vi "RPi_I2C_BME280_read_example.vi"() -> ()   [LabVIEW 2020]
doc: "This example shows how to read the BMP280 sensor by using a Raspberry PI and LabVIEW.\n\nMIT License\nCopyright (c) 2021 Asper"
uses:
  <vilib>/MakerHub/LINX/Public/Utilities/Open Local.vi
  <vilib>/MakerHub/LINX/LMH-LINX.lvlib
panel:
  out "Graph":T1(graph)
  in  "Stop":bool
  out "Last measures":T2
  out "Error Out":errorcluster
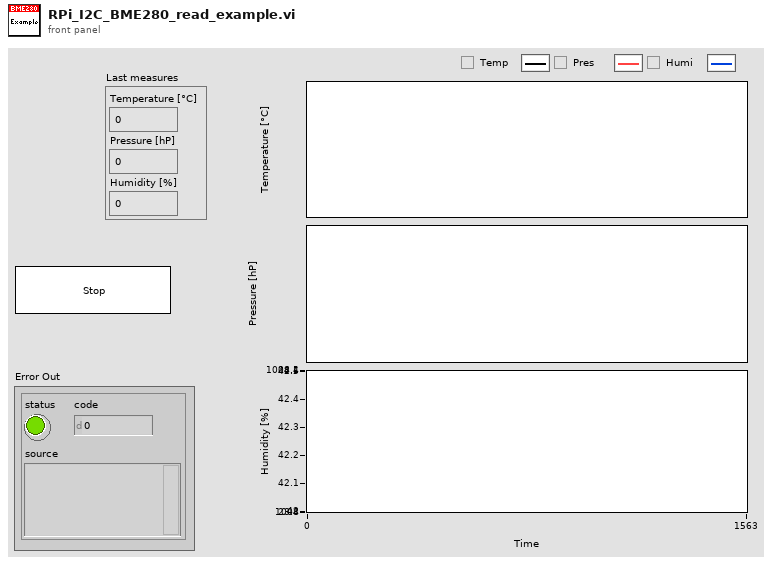
[diagram p1: front panel]
types:
  T1 = cluster{"Temperature":dbl, "Pressure":dbl, "Humidity":dbl}
  T2 = cluster{"Temperature [°C]":dbl, "Pressure [hP]":dbl, "Humidity [%]":dbl}
  T3 = typedef "LMH-LINX.lvlib/LINX Ref.ctl" = cluster{"IO":T4, "Interface":T5, "LINX Device Config":T6}
  T4 = typedef "LMH-LINX.lvlib/Platform.ctl" = enum16{"Remote", "Local"}
  T5 = typedef "LMH-LINX.lvlib/Interface.ctl" = enum16{"Serial", "TCP"}
  T6 = typedef "LMH-LINX.lvlib/Device.lvlib/LINX Device Config.ctl" = cluster{"Interface":T5, "COM Port":refnum<visa-resource-name>, "TCP Configuration":T7, "Device Family":u8, "Device ID":u8, "Device Name":string, "TCP Ref":refnum<k5>, "Channels":T8}
  T7 = typedef "LMH-LINX.lvlib/Device.lvlib/TCP Config.ctl" = cluster{"IP Address":string, "Port":u16}
  T8 = typedef "LMH-LINX.lvlib/Channels.ctl" = cluster{"DI":u8[], "DO":u8[], "AI":u8[], "AO":u8[], "PWM":u8[], "QE":u8[], "UART":u8[], "I2C 2":u8[], "SPI":u8[], "CAN":u8[], "Servo":u8[], "AI Ref (V)":dbl, "AI Resolution (Bits)":u8, "AO Ref (V)":dbl, "AO Resolution (Bits)":u8}
  T9 = typedef "BME280_Calibration_Coefficients.ctl" = cluster{"Temperature":cluster{"dig_T1":u16, "dig_T2":i16, "dig_T3":i16}, "Pressure":cluster{"dig_P1":u16, "dig_P2":i16, "dig_P3":i16, "dig_P4":i16, "dig_P5":i16, "dig_P6":i16, "dig_P7":i16, "dig_P8":i16, "dig_P9":i16}, "Humidity":cluster{"dig_H1":u8, "dig_H2":i16, "dig_H3":u8, "dig_H4":i16, "dig_H5":i16, "dig_H6":i8}}
  T10 = cluster{"pres_raw":u32, "temp_raw":u32, "hum_raw":u32}
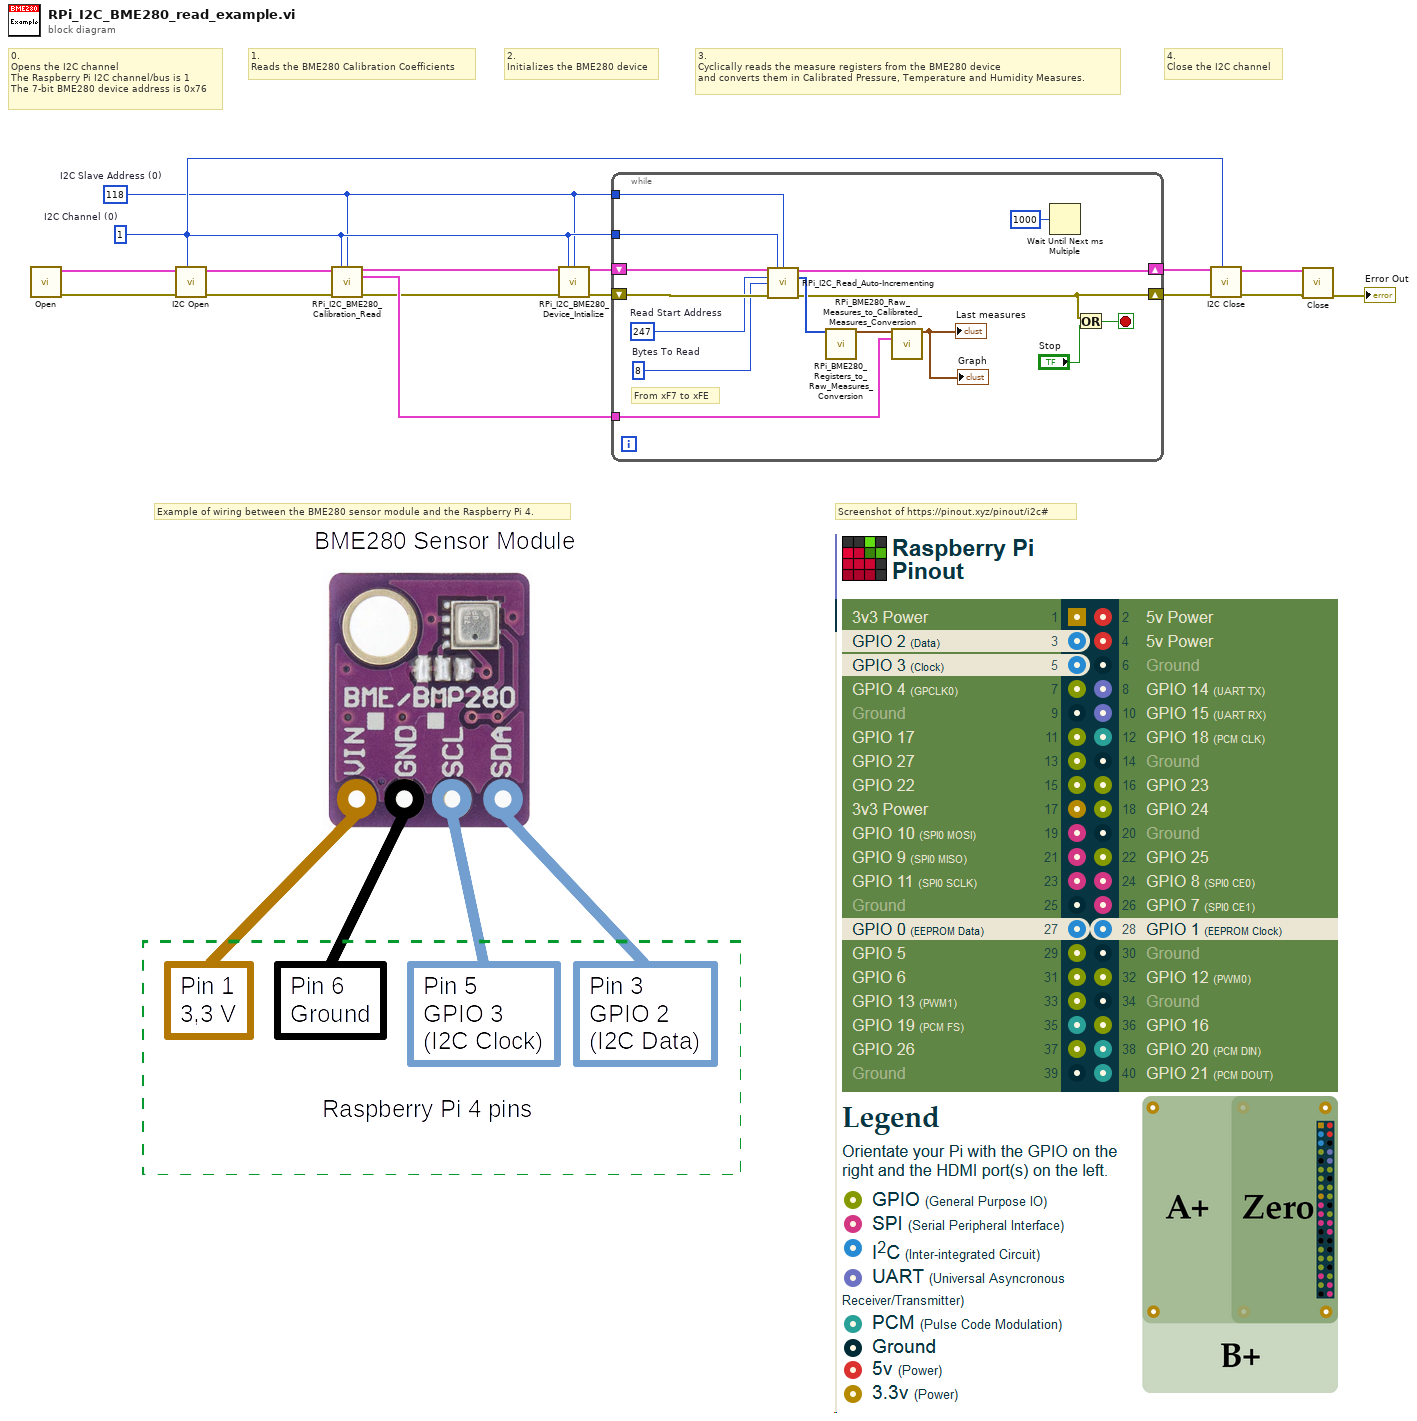
[diagram p0: block diagram]
diagram:
  w2 = u8 1  # I2C Channel (0)
  w1 = u8 118  # I2C Slave Address (0)
  # "Example of wiring between the BME280 sensor module and the Raspberry Pi 4."
  # "Screenshot of https://pinout.xyz/pinout/i2c#"
  # "4.\nClose the I2C channel"
  # "0.\nOpens the I2C channel\nThe Raspberry Pi I2C channel/bus is 1\nThe 7-bit BME280 device address is 0x76"
  # "1.\nReads the BME280 Calibration Coefficients"
  # "3.\nCyclically reads the measure registers from the BME280 device\nand converts them in Calibrated Pressure, Temperature and Humidity Measures."
  # "2.\nInitializes the BME280 device"
  n1 = call-poly <vilib>:"Open.vi"() -> ("Error Out"=w15:errorcluster, "LINX Resource"=w16:T3)  [unwired: 9 in, 1 out]
  n2 = call <vilib>:"I2C Open.vi"("I2C Channel (0)"=w2, "Error In"=w15, "LINX Resource"=w16) -> ("Error Out"=w5:errorcluster, "LINX Resource"=w6:T3)  [unwired: 7 in]
  n3 = call "RPi_I2C_BME280_Calibration_Read.vi"("LINX Resource"=w6, "I2C Channel (0)"=w2, "I2C Slave Address (0)"=w1, "error in (no error)"=w5) -> ("LINX Resource out"=w4:T3, "Calibration Coefficients"=w7:T9, "error out"=w3:errorcluster)  [unwired: 9 in]
  n4 = call "RPi_I2C_BME280_Device_Intialize.vi"("LINX Resource in"=w4, "I2C Channel (0)"=w2, "I2C Slave Address (0)"=w1, "error in (no error)"=w3) -> ("LINX Resource out"=w11:T3, "error out"=w10:errorcluster)  [unwired: 10 in]
  n5 = while {
    tunnel: w1 -> [w21]
    tunnel: w2 -> [w20]
    tunnel: w7 -> [w30]
    shift-right: [w18] -> w9
    shift-left: w11 -> [w25]
    shift-right: [w17] -> w8
    shift-left: w10 -> [w24]
    stop <- w29 stop-if-true
    w23 = u8 247  # Read Start Address
    w22 = u8 8  # Bytes To Read
    # "From xF7 to xFE"
    n6 = call "RPi_I2C_Read_Auto-Incrementing.vi"("LINX Resource in"=w25, "I2C Channel (0)"=w20, "I2C Slave Address (0)"=w21, "Start Register Address"=w23, "Number of Bytes To Read"=w22, "error in (no error)"=w24) -> ("LINX Resource out"=w18:T3, "Registers (Bytes)"=w19:u8[], "error out"=w17:errorcluster)  [unwired: 7 in]
    n7 = call "RPi_BME280_Registers_to_Raw_Measures_Conversion.vi"("Registers (Bytes)"=w19) -> ("Raw Measures"=w31:T10)  [unwired: 14 in]
    n8 = call "RPi_BME280_Raw_Measures_to_Calibrated_Measures_Conversion.vi"("Raw Measures"=w31, "Calibration Coefficients"=w30) -> ("Calibrated Measures"=→"Last measures" →"Graph":T1)  [unwired: 13 in]
    n9 = Wait Until Next ms Multiple(millisecond multiple=u32 1000) -> ()  [unwired: 1 out]
    n10 = Or(x=w17, y="Stop") -> (x .or. y?=w29:bool)
  }
  n11 = call <vilib>:"I2C Close.vi"("I2C Channel (0)"=w2, "Error In"=w8, "LINX Resource"=w9) -> ("Error Out"=w14:errorcluster, "LINX Resource"=w13:T3)  [unwired: 7 in]
  n12 = call <vilib>:"Close.vi"("Error In"=w14, "LINX Resource"=w13) -> ("Error Out"=→"Error Out":errorcluster)  [unwired: 9 in]
